vi "Configure Reference Oscillator.vi"(8 "error in (no error)":errorcluster, 9 "Source Auto Selection(T: Enable)":bool=TRUE, 10 "Source (0: Internal)":i32(ring) items=["Internal", "External"], 11 "VISA resource name":refnum<visa-resource-name>) -> (0 "error out":errorcluster, 3 "VISA resource name out":refnum<visa-resource-name>)   [LabVIEW 2017, in "Agilent 3352X Series.lvlib"]
doc: "Controls the Reference Oscillator subsystem use of the 10 MHz reference oscillator and the External Reference oscillator input. The Reference Oscillator serves as the primary clock signal to control all waveform synthesis in the instrument.\nUse this VI to select the reference oscillator signal used as a frequency/phase reference for the instrument.\n\n<b>Note</b>:\nOnly Valid when the instrument contains the optional OCXO oscillator. \nNot applicable for EDU33211A and EDU33212A models."
uses:
  Doppia_Freq_Circuito/Agilent 3352X Series/Agilent 3352X Series.lvlib
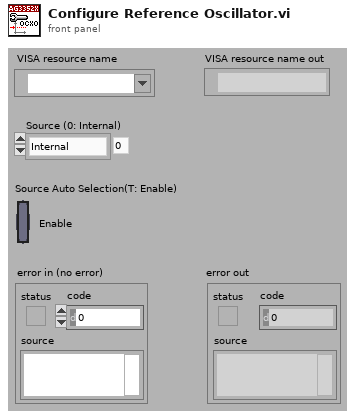
[diagram p1: front panel]
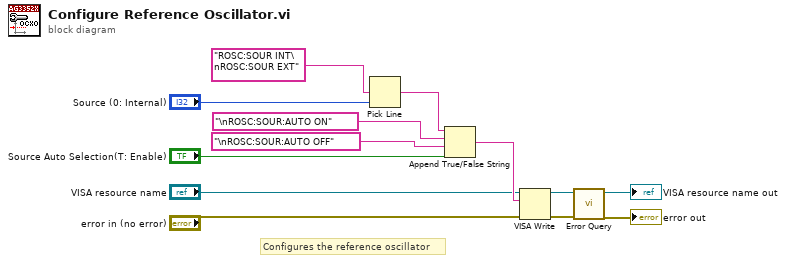
[diagram p0: block diagram]
diagram:
  # "Configures the reference oscillator"
  n1 = Pick Line(multi-line string="ROSC:SOUR INT\nROSC:SOUR EXT", line index="Source (0: Internal)") -> (output string=w11:string)  [unwired: 1 out]
  n2 = Append True/False String(1:"Source Auto Selection(T: Enable)", 2:"\nROSC:SOUR:AUTO OFF", 3:"\nROSC:SOUR:AUTO ON", 4:w11) -> (0:w7:string)
  n3 = VISA Write(VISA resource name="VISA resource name", write buffer=w7, error in (no error)="error in (no error)") -> (VISA resource name out=w4:refnum<visa-resource-name>, error out=w3:errorcluster)  [unwired: 1 out]
  n4 = call "Error Query.vi"("error in (no error)"=w3, "VISA resource name"=w4) -> ("error out"=→"error out":errorcluster, "VISA resource name out"=→"VISA resource name out":refnum<visa-resource-name>)  [unwired: 8 out]
